vi "DrawLine2.vi"(1 "Color":u32(colorbox)=16711680, 2 "输入簇":T1, 3 "img in":T2) -> (0 "Image Out":T2)   [LabVIEW 2014]
uses:
  <vilib>/vision/Image Controls.llb/IMAQ Image.ctl
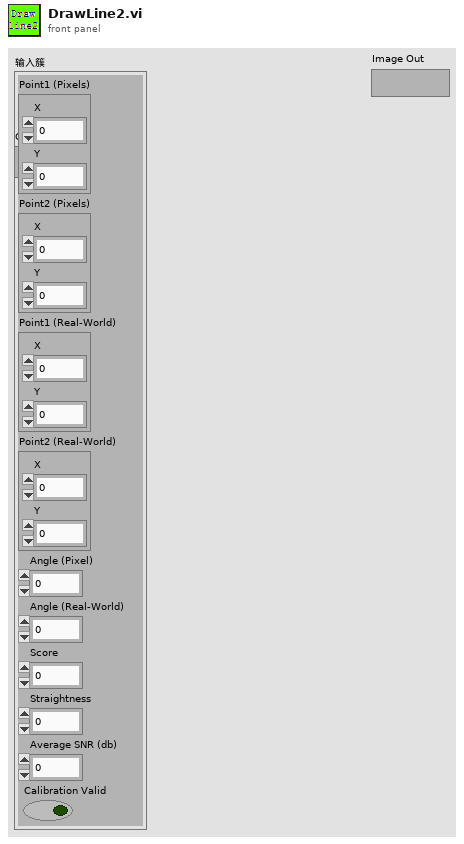
[diagram p1: front panel]
types:
  T1 = cluster{"Point1 (Pixels)":cluster{"X":sgl, "Y":sgl}, "Point2 (Pixels)":cluster{"X":sgl, "Y":sgl}, "Point1 (Real-World)":cluster{"X":sgl, "Y":sgl}, "Point2 (Real-World)":cluster{"X":sgl, "Y":sgl}, "Angle (Pixel)":dbl, "Angle (Real-World)":dbl, "Score":dbl, "Straightness":dbl, "Average SNR (db)":dbl, "Calibration Valid":bool}
  T2 = typedef "IMAQ Image.ctl" = refnum<image>
  T3 = cluster{"Point1 (Pixels)":cluster{"X":sgl, "Y":sgl}, "Point2 (Pixels)":cluster{"X":sgl, "Y":sgl}}
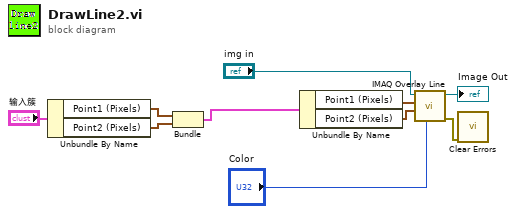
[diagram p0: block diagram]
diagram:
  n1 = Unbundle By Name("输入簇") -> ("Point1 (Pixels)"=w4:cluster{"X":sgl, "Y":sgl}, "Point2 (Pixels)"=w3:cluster{"X":sgl, "Y":sgl})
  n2 = Bundle("Point1 (Pixels)"=w4, "Point2 (Pixels)"=w3) -> (w2:T3)  [unwired: 1 in]
  n3 = Unbundle By Name(w2) -> ("Point1 (Pixels)"=w8:cluster{"X":sgl, "Y":sgl}, "Point2 (Pixels)"=w9:cluster{"X":sgl, "Y":sgl})
  n4 = call "IMAQ Overlay Line"("Color"="Color", "End Point"=w9, "Start Point"=w8, "Image"="img in") -> ("error out"=w5:errorcluster, "Image Out"=→"Image Out":T2)  [unwired: 6 in]
  n5 = call <vilib>:"Clear Errors.vi"("error in (no error)"=w5) -> ()  [unwired: 5 in, 2 out]
